vi "Recibir_Solicitud_Movimiento.vi"(8 "error in (no error)":errorcluster, 9 "Distancia":T1 items=["10cm"=9100, "1cm"=910, "1mm"=91, "0.1mm"=9, "1 paso "=1], 10 "Enum":T2, 11 "VISA resource name":refnum<visa-resource-name>) -> (0 "error out":errorcluster)   [LabVIEW 2019]
uses:
  Typedefs/Tipo_movimiento.ctl
  Typedefs/Distancia.ctl
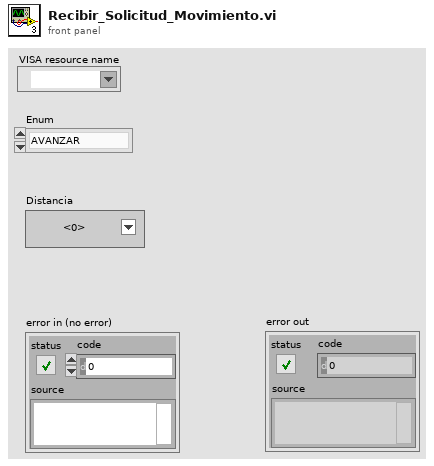
[diagram p1: front panel]
types:
  T1 = typedef "Distancia.ctl" = i16
  T2 = typedef "Tipo_movimiento.ctl" = enum16{"AVANZAR", "RETROCEDER", "DERECHA", "IZQUIERDA", "SUBIRZ", "BAJARZ", "POSICION INICIO"}
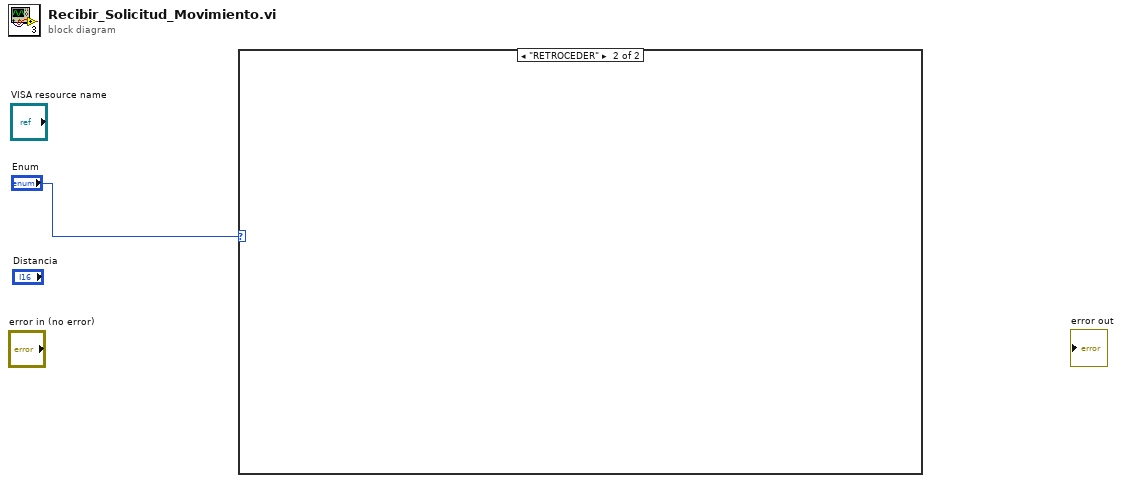
[diagram p0: block diagram]
diagram:
  n1 = case shown="\"RETROCEDER\"" "Enum" {
    frame "AVANZAR", Default {
    }
    frame "RETROCEDER" {
    }
  }
